vi "Get_AOI_size&position.vi"(7 "error in (no error)":errorcluster, 10 ".NET Refnum in":refnum<k24>) -> (0 "error out":errorcluster, 1 "s32Height":i32, 2 "s32Width":i32, 3 ".NET Refnum out":refnum<k24>)   [LabVIEW 2021]
uses:
  C:/Program Files/Thorlabs/Scientific Imaging/ThorCam/uc480DotNet.dll
  Program Files/Thorlabs/Scientific Imaging/ThorCam/uc480DotNet.dll
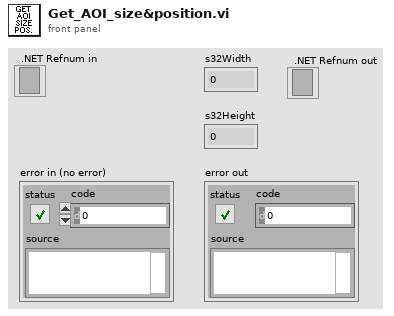
[diagram p1: front panel]
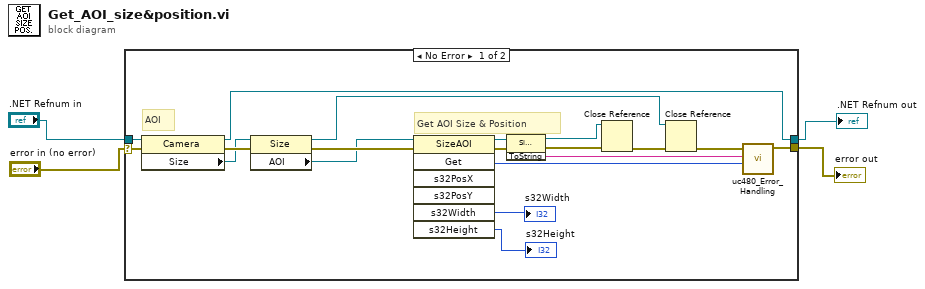
[diagram p0: block diagram]
diagram:
  n1 = case shown="No Error" "error in (no error)" {
    selector: "error in (no error)" -> [w6 w25]
    tunnel: ".NET Refnum in" -> [w23 w24]
    tunnel: [w13 w25] -> w3
    tunnel: [w5 w24] -> w1
    frame No Error {
      # "Get AOI Size & Position"
      # "AOI"
      n2 = property class="Camera"(reference=w23, error in=w6) -> (reference out=w5:refnum<k24>, error out=w8:errorcluster, "Size"=w7:refnum<k24>)
      n3 = property class="Size"(reference=w7, error in=w8) -> (reference out=w22:refnum<k24>, error out=w17:errorcluster, "AOI"=w16:refnum<k24>)
      n4 = invoke class="SizeAOI" method="Get"(reference=w16, error in=w17) -> (reference out=w10:refnum<k24>, error out=w11:errorcluster, "Get"=w12:i32, "s32Width"=→"s32Width":i32, "s32Height"=→"s32Height":i32)  [unwired: 5 in, 2 out]
      n5 = invoke class="SizeAOI" method="ToString"(reference=w10, error in=w11) -> (reference out=w19:refnum<k24>, error out=w18:errorcluster, "ToString"=w9:string)  [unwired: 1 in]
      n6 = Close Reference(reference=w19, error in (no error)=w18) -> (error out=w20:errorcluster)
      n7 = Close Reference(reference=w22, error in (no error)=w20) -> (error out=w21:errorcluster)
      n8 = call "uc480_Error_Handling.vi"("Error Code"=w12, "Error String"=w9, "Error In"=w21) -> ("Error Out"=w13:errorcluster)  [unwired: 8 in]
    }
    frame Error {
    }
  }
  "error out" <- w3
  ".NET Refnum out" <- w1
